vi "Trama_Serial_DAQ.vi"(3 "error in (no error)":errorcluster, 4 "memoria_trama":string, 5 "reference":refnum<visa-resource-name>) -> (0 "error out":errorcluster, 1 "Trama_Out":string, 2 "reference 2":refnum<visa-resource-name>)   [LabVIEW 2019]
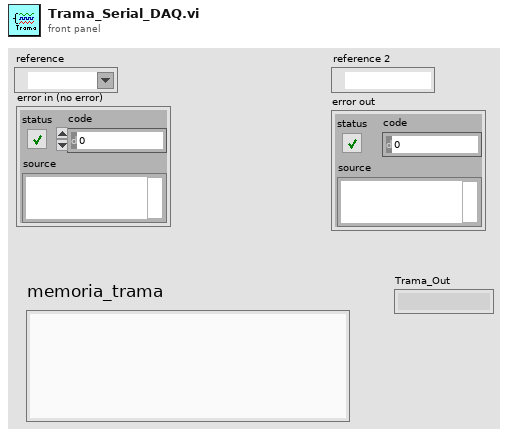
[diagram p1: front panel]
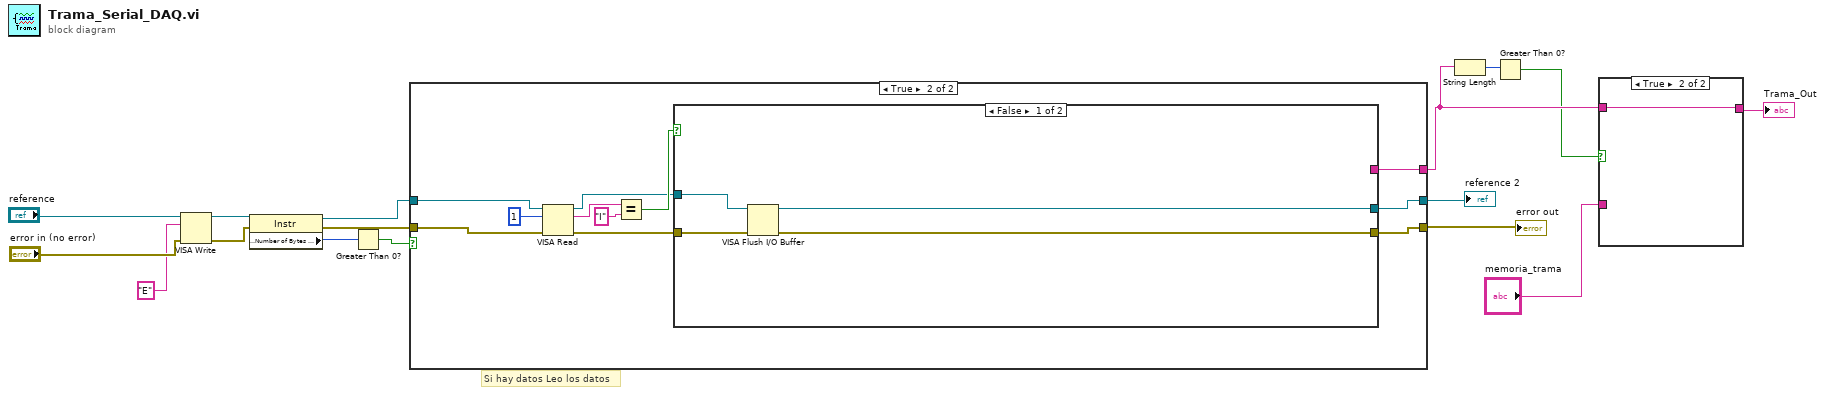
[diagram p0: block diagram]
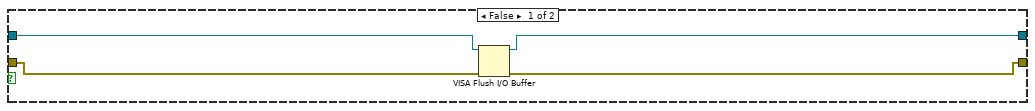
[diagram p3: hidden frame]
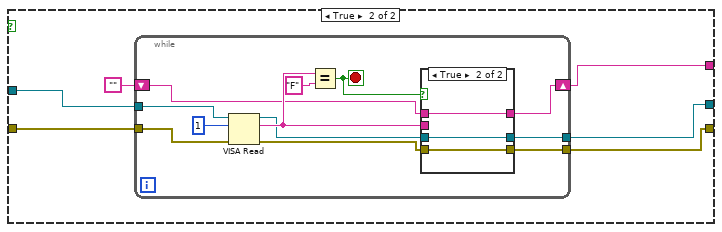
[diagram p4: hidden frame]
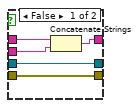
[diagram p5: hidden frame]
diagram:
  # "Si hay datos Leo los datos"
  n1 = VISA Write(VISA resource name="reference", write buffer="E", error in (no error)="error in (no error)") -> (VISA resource name out=w5:refnum<visa-resource-name>, error out=w4:errorcluster)  [unwired: 1 out]
  n2 = property class="Instr"(reference=w5, error in=w4) -> (reference out=w13:refnum<visa-resource-name>, error out=w16:errorcluster, "Serial Settings:Number of Bytes at Serial Port"=w15:u32)
  n3 = Greater Than 0?(x=w15) -> (x > 0?=w14:bool)
  n4 = case shown="True" w14 {
    tunnel: [w18 w25] -> w12
    tunnel: [w17 w24] -> w11
    tunnel: w13 -> [w20 w23]
    tunnel: w16 -> [w19 w22]
    tunnel: [_ w21] -> w8
    frame False {
      n5 = VISA Flush I/O Buffer(VISA resource name=w20, error in (no error)=w19) -> (VISA resource name out=w18:refnum<visa-resource-name>, error out=w17:errorcluster)  [unwired: 1 in]
    }
    frame True {
      n6 = VISA Read(VISA resource name=w23, byte count=u32 1, error in (no error)=w22) -> (VISA resource name out=w27:refnum<visa-resource-name>, read buffer=w30:string, error out=w26:errorcluster)  [unwired: 1 out]
      n7 = Equal?(x=w30, y="I") -> (x = y?=w28:bool)
      n8 = case shown="False" w28 {
        tunnel: w27 -> [w35 w41]
        tunnel: w26 -> [w34 w40]
        tunnel: [w33 w38] -> w25
        tunnel: [w32 w37] -> w24
        tunnel: [_ w36] -> w21
        frame False {
          n9 = VISA Flush I/O Buffer(VISA resource name=w35, error in (no error)=w34) -> (VISA resource name out=w33:refnum<visa-resource-name>, error out=w32:errorcluster)  [unwired: 1 in]
        }
        frame True {
          n10 = while {
            tunnel: w41 -> [w53]
            tunnel: w40 -> [w52]
            shift-right: [w46] -> w36
            shift-left: "" -> [w47]
            tunnel: [w44] -> w38
            tunnel: [w43] -> w37
            stop <- w49 stop-if-true
            n11 = VISA Read(VISA resource name=w53, byte count=u32 1, error in (no error)=w52) -> (VISA resource name out=w45:refnum<visa-resource-name>, read buffer=w48:string, error out=w42:errorcluster)  [unwired: 1 out]
            n12 = Equal?(x=w48, y="F") -> (x = y?=w49:bool)
            n13 = case shown="True" w49 {
              tunnel: w48 -> [w55 _]
              tunnel: w47 -> [w56 w59]
              tunnel: [w54 w59] -> w46
              tunnel: [w58 w61] -> w44
              tunnel: w45 -> [w58 w61]
              tunnel: [w57 w60] -> w43
              tunnel: w42 -> [w57 w60]
              frame False {
                n14 = Concatenate Strings(w56, w55) -> (w54:string)
              }
              frame True {
              }
            }
          }
        }
      }
    }
  }
  "reference 2" <- w12
  "error out" <- w11
  n15 = String Length(string=w8) -> (length=w7:i32)
  n16 = Greater Than 0?(x=w7) -> (x > 0?=w6:bool)
  n17 = case shown="True" w6 {
    tunnel: [w62 w63] -> w9
    tunnel: w8 -> [_ w63]
    tunnel: "memoria_trama" -> [w62 _]
    frame False {
    }
    frame True {
    }
  }
  "Trama_Out" <- w9
